vi "Practica03.vi"() -> ()   [LabVIEW 2020]
panel:
  in  "stop":bool
  out "Value":bool
  in  "ValorMenor":dbl=25.0
  in  "ValorMayor":dbl=27.0
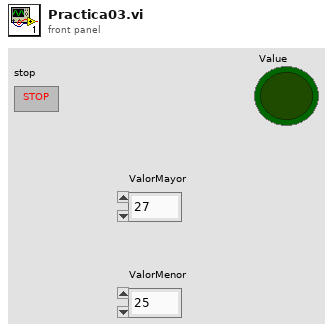
[diagram p1: front panel]
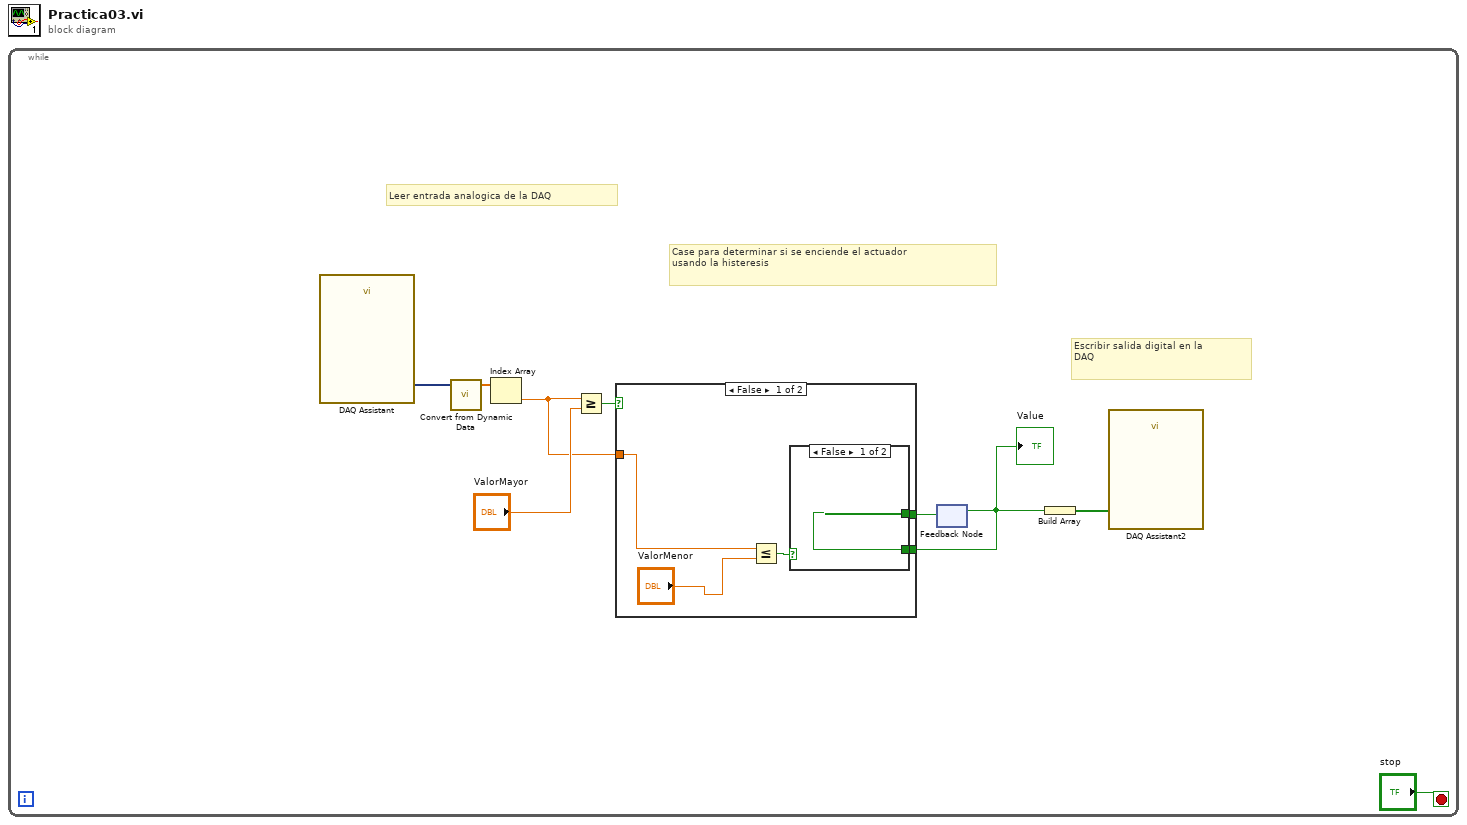
[diagram p0: block diagram]
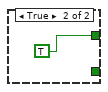
[diagram p2: hidden frame]
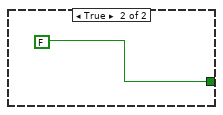
[diagram p3: hidden frame]
diagram:
  n1 = while {
    stop <- "stop" stop-if-true
    # "Escribir salida digital en la\nDAQ"
    # "Case para determinar si se enciende el actuador \nusando la histeresis"
    # "Leer entrada analogica de la DAQ"
    n2 = call "DAQ Assistant"() -> ("data"=w5:dynamicdata)  [unwired: 17 in, 2 out]
    n3 = call "Convert from Dynamic Data"("Dynamic Data Type"=w5) -> ("Array"=w3:dbl[])  [unwired: 3 in]
    n4 = Index Array(array=w3) -> (element=w4:dbl)  [unwired: 1 in]
    n5 = Greater Or Equal?(x=w4, y="ValorMayor") -> (x >= y?=w8:bool)
    n6 = feedback #1() -> (w2:bool)  [unwired: 1 in]
    "Value" <- w2
    n7 = case shown="False" w8 {
      tunnel: w4 -> [w14 _]
      tunnel: [w12 FALSE] -> w9
      tunnel: w2 -> [w10 _]
      frame False {
        n8 = Less Or Equal?(x=w14, y="ValorMenor") -> (x <= y?=w13:bool)
        n9 = case shown="False" w13 {
          tunnel: [w15 TRUE] -> w12
          tunnel: w10 -> [w15 _]
          frame False {
          }
          frame True {
          }
        }
      }
      frame True {
      }
    }
    n10 = feedback-in #1(w9) -> ()
    n11 = Build Array(w2) -> (w1:bool[])
    n12 = call "DAQ Assistant2"("data"=w1) -> ()  [unwired: 17 in, 2 out]
  }
